vi "Parse Parameters File.vi"(8 "error in":errorcluster, 11 "path to XML document":path caption="path to parameters xml") -> (0 "error out":errorcluster, 2 "biu configuration":T1, 3 "path to XML document out":path caption="path to parameters xml")   [LabVIEW 2020, in "MIL-STD 1553 Import.lvlib"]
uses:
  MIL-STD 1553 Import.lvlib
  Shared/BIU Configuration.ctl
  Shared/Address.ctl
  Shared/Major Frame Definition.ctl
  Shared/Minor Frame Definition.ctl
  Shared/Acyclic Frame Definition.ctl
  Shared/Message Definition.ctl
  Shared/Message Type.ctl
  Shared/Terminal Endpoint.ctl
  Shared/Parameter Definition.ctl
  a98a4505-1d2b-4178-8eef-924facff6c40.vi
  60cc2e63-67cc-4215-8c07-088d80cb97fe.vi
  a98a4505-1d2b-4178-8eef-924facff6c40.vi/b1e6fcf8-dac1-42d2-b1fe-151afe06dbd4.vi
  60cc2e63-67cc-4215-8c07-088d80cb97fe.vi/b1e6fcf8-dac1-42d2-b1fe-151afe06dbd4.vi
  a98a4505-1d2b-4178-8eef-924facff6c40.vi/b1e6fcf8-dac1-42d2-b1fe-151afe06dbd4.vi/49c1b1ee-2d2a-4a85-8ca5-42123c34e85a.vi
  60cc2e63-67cc-4215-8c07-088d80cb97fe.vi/b1e6fcf8-dac1-42d2-b1fe-151afe06dbd4.vi/49c1b1ee-2d2a-4a85-8ca5-42123c34e85a.vi
  <vilib>/xml/Load XML File.vi
  Constants.vi
  <vilib>/xml/Get Node Text Content.vi
  <vilib>/Utility/error.llb/Error Cluster From Error Code.vi
  <vilib>/xml/Close Reference(Node).vi
  <vilib>/Utility/xml.llb/Write to XML File(string).vi
  <resource>/objmgr/DOMUserDefRef.rc
  <vilib>/xml/NI_XML.lvlib
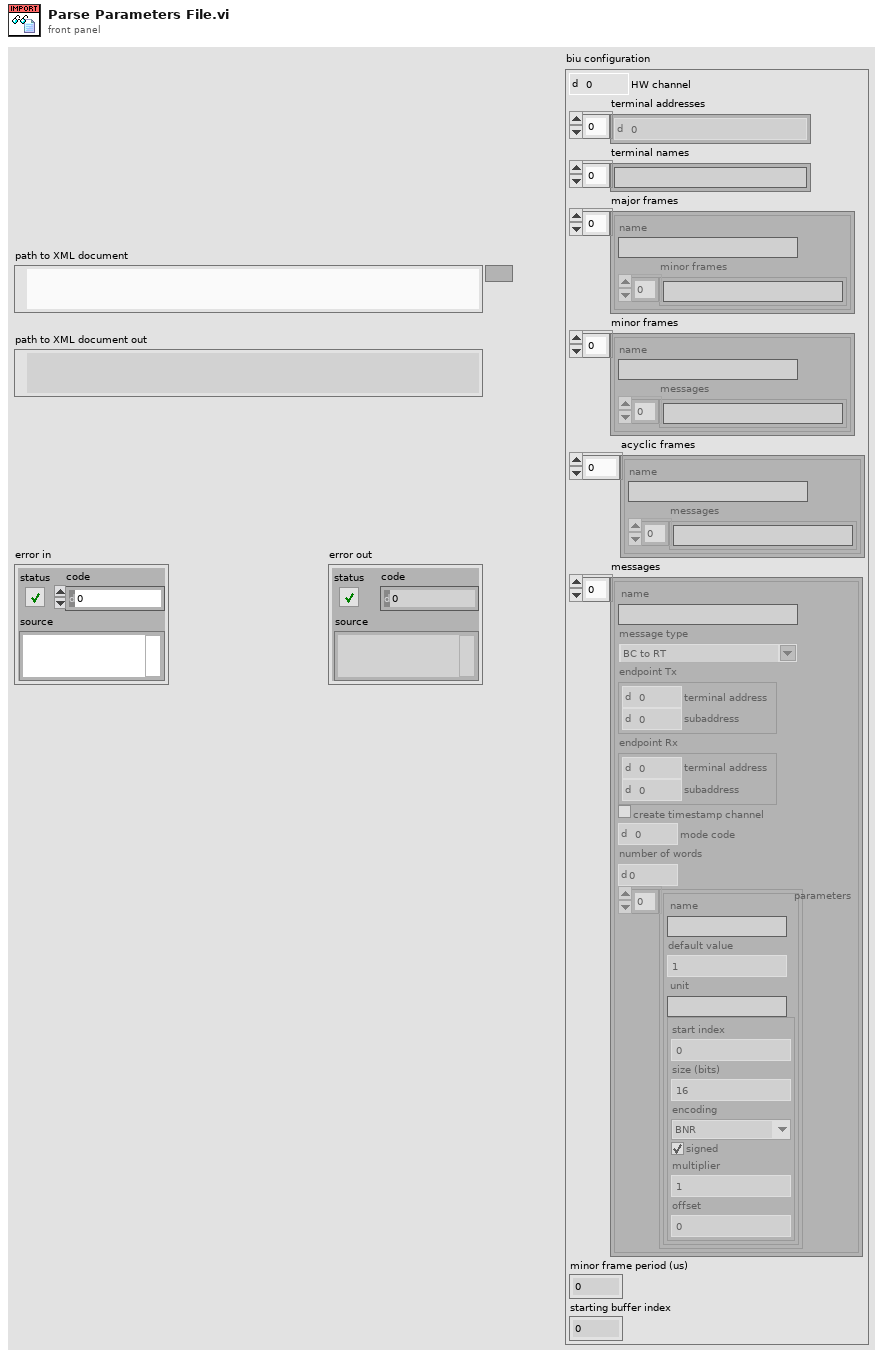
[diagram p1: front panel]
types:
  T1 = typedef "BIU Configuration.ctl" = cluster{"HW channel":u16, "terminal addresses":T2[], "terminal names":string[], "major frames":T3[], "minor frames":T4[], "acyclic frames":T5[], "messages":T6[], "minor frame period (us)":i32, "starting buffer index":u16}
  T2 = typedef "Address.ctl" = u16
  T3 = typedef "Major Frame Definition.ctl" = cluster{"name":string, "minor frames":string[]}
  T4 = typedef "Minor Frame Definition.ctl" = cluster{"name":string, "messages":string[]}
  T5 = typedef "Acyclic Frame Definition.ctl" = cluster{"name":string, "messages":string[]}
  T6 = typedef "Message Definition.ctl" = cluster{"name":string, "message type":T7, "endpoint Tx":T8, "endpoint Rx":T8, "create timestamp channel":bool, "mode code":u16, "number of words":u16, "parameters":cluster{"name":string, "default value":dbl, "unit":string, "parameter definition":T9}[]}
  T7 = typedef "Message Type.ctl" = string
  T8 = typedef "Terminal Endpoint.ctl" = cluster{"terminal address":T2, "subaddress":T2}
  T9 = typedef "Parameter Definition.ctl" = cluster{"start index":i32, "size (bits)":i32, "encoding":enum16{"BNR", "BCD", "Discrete"}, "signed":bool, "multiplier":dbl, "offset":dbl}
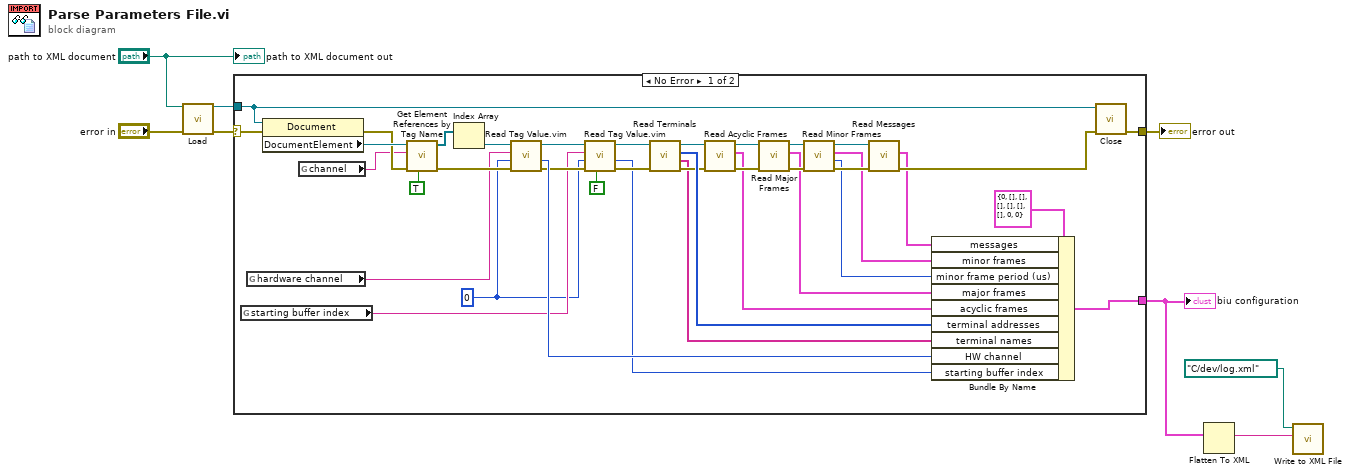
[diagram p0: block diagram]
diagram:
  n1 = call-poly <vilib>:"Load.vi"("path to XML document"="path to XML document", "error in (no error)"="error in") -> ("DOM document out"=w5:refnum<k20>, "error out"=w8:errorcluster)  [unwired: 11 in, 1 out]
  n2 = case shown="No Error" w8 {
    selector: w8 -> [w46 w47]
    tunnel: [w45 w47] -> w6
    tunnel: w5 -> [w44 _]
    tunnel: [w37 _] -> w3
    frame No Error {
      w9 = u16 0
      n3 = global read "Constants.vi" "starting buffer index"() -> (w11:string)
      n4 = global read "Constants.vi" "hardware channel"() -> (w38:string)
      n5 = property class="Document"(reference=w44, error in=w46) -> (error out=w42:errorcluster, "DocumentElement"=w43:refnum<k20>)  [unwired: 1 out]
      n6 = global read "Constants.vi" "channel"() -> (w41:string)
      n7 = call "Get Element References by Tag Name.vi"("required (F)"=TRUE, "error in"=w42, "tag name"=w41, "node in"=w43) -> ("error out"=w40:errorcluster, "array of elements"=w33:refnum<k20>[])  [unwired: 6 in]
      n8 = Index Array(array=w33) -> (element=w34:refnum<k20>)  [unwired: 1 in]
      n9 = call "Read Tag Value.vim"("error in"=w40, "default"=w9, "tag name"=w38, "node in"=w34) -> ("error out"=w16:errorcluster, "value"=w32:u16, "node out"=w15:refnum<k20>)  [unwired: 5 in]
      n10 = call "Read Tag Value.vim"("required (F)"=FALSE, "error in"=w16, "default"=w9, "tag name"=w11, "node in"=w15) -> ("error out"=w13:errorcluster, "value"=w10:u16, "node out"=w14:refnum<k20>)  [unwired: 4 in]
      n11 = call "Read Terminals.vi"("error in"=w13, "channel ref in"=w14) -> ("error out"=w29:errorcluster, "terminal names"=w28:string[], "terminal addresses"=w31:T2[], "channel ref out"=w30:refnum<k20>)  [unwired: 6 in]
      n12 = call "Read Acyclic Frames.vi"("error in"=w29, "channel ref in"=w30) -> ("error out"=w23:errorcluster, "acyclic frames"=w18:T5[], "channel ref out"=w25:refnum<k20>)  [unwired: 7 in]
      n13 = call "Read Major Frames.vi"("error in"=w23, "channel ref in"=w25) -> ("error out"=w22:errorcluster, "major frames"=w19:T3[], "channel ref out"=w24:refnum<k20>)  [unwired: 7 in]
      n14 = call "Read Minor Frames.vi"("error in"=w22, "channel ref in"=w24) -> ("error out"=w26:errorcluster, "minor frame period (us)"=w17:i32, "minor frames"=w20:T4[], "channel ref out"=w27:refnum<k20>)  [unwired: 6 in]
      n15 = call "Read Messages.vi"("error in"=w26, "channel ref in"=w27) -> ("error out"=w36:errorcluster, "messages"=w21:T6[])  [unwired: 7 in, 1 out]
      n16 = Bundle By Name(cluster=T1 {"HW channel"=0, "terminal addresses"=[], "terminal names"=[], "major frames"=[], "minor frames"=[], "acyclic frames"=[], "messages"=[], "minor frame period (us)"=0, "starting buffer index"=0} ("1553 channel"), "messages"=w21, "minor frames"=w20, "minor frame period (us)"=w17, "major frames"=w19, "acyclic frames"=w18, "terminal addresses"=w31, "terminal names"=w28, "HW channel"=w32, "starting buffer index"=w10) -> (w37:T1)
      n17 = call-poly <vilib>:"Close.vi"("error in (no error)"=w36, "node"=w44) -> ("error out"=w45:errorcluster)  [unwired: 7 in]
    }
    frame Error {
    }
  }
  "error out" <- w6
  "biu configuration" <- w3
  n18 = Flatten To XML(6:w3) -> (2:w1:string)
  n19 = call-poly <vilib>:"Write to XML File.vi"("XML Input"=w1, "XML File Path"=path "C:/dev/log.xml") -> ()  [unwired: 7 in, 3 out]
  "path to XML document out" <- "path to XML document"
